vi "Read.vi"(8 "error in (no error)":errorcluster, 11 "Keyboard in":refnum<class "Keyboard.lvclass">) -> (0 "error out":errorcluster, 1 "Velocity out":dbl, 2 "Direction out":cluster{dbl, dbl}, 4 "Stop?":bool, 5 "Boost?":bool)   [LabVIEW 2024, in "Keyboard.lvclass"]
doc: "MIT Licence\nCopyright (c) 2024 David Grollier"
uses:
  Keyboard.lvclass
  Input Device.lvclass/Input Device.ctl
  Keyboard.lvclass/Keyboard.ctl
  <vilib>/Utility/error.llb/Error Cluster From Error Code.vi
  <vilib>/ErrorRing/Error Ring.xnode
  Input Device.lvclass
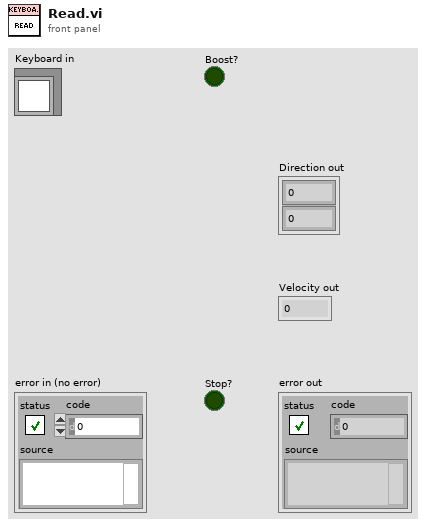
[diagram p1: front panel]
types:
  T1 = cluster{"Keyboard Registration Refnum":refnum<event-registration>, "Stop Event Registration Refnum out":refnum<event-registration>}
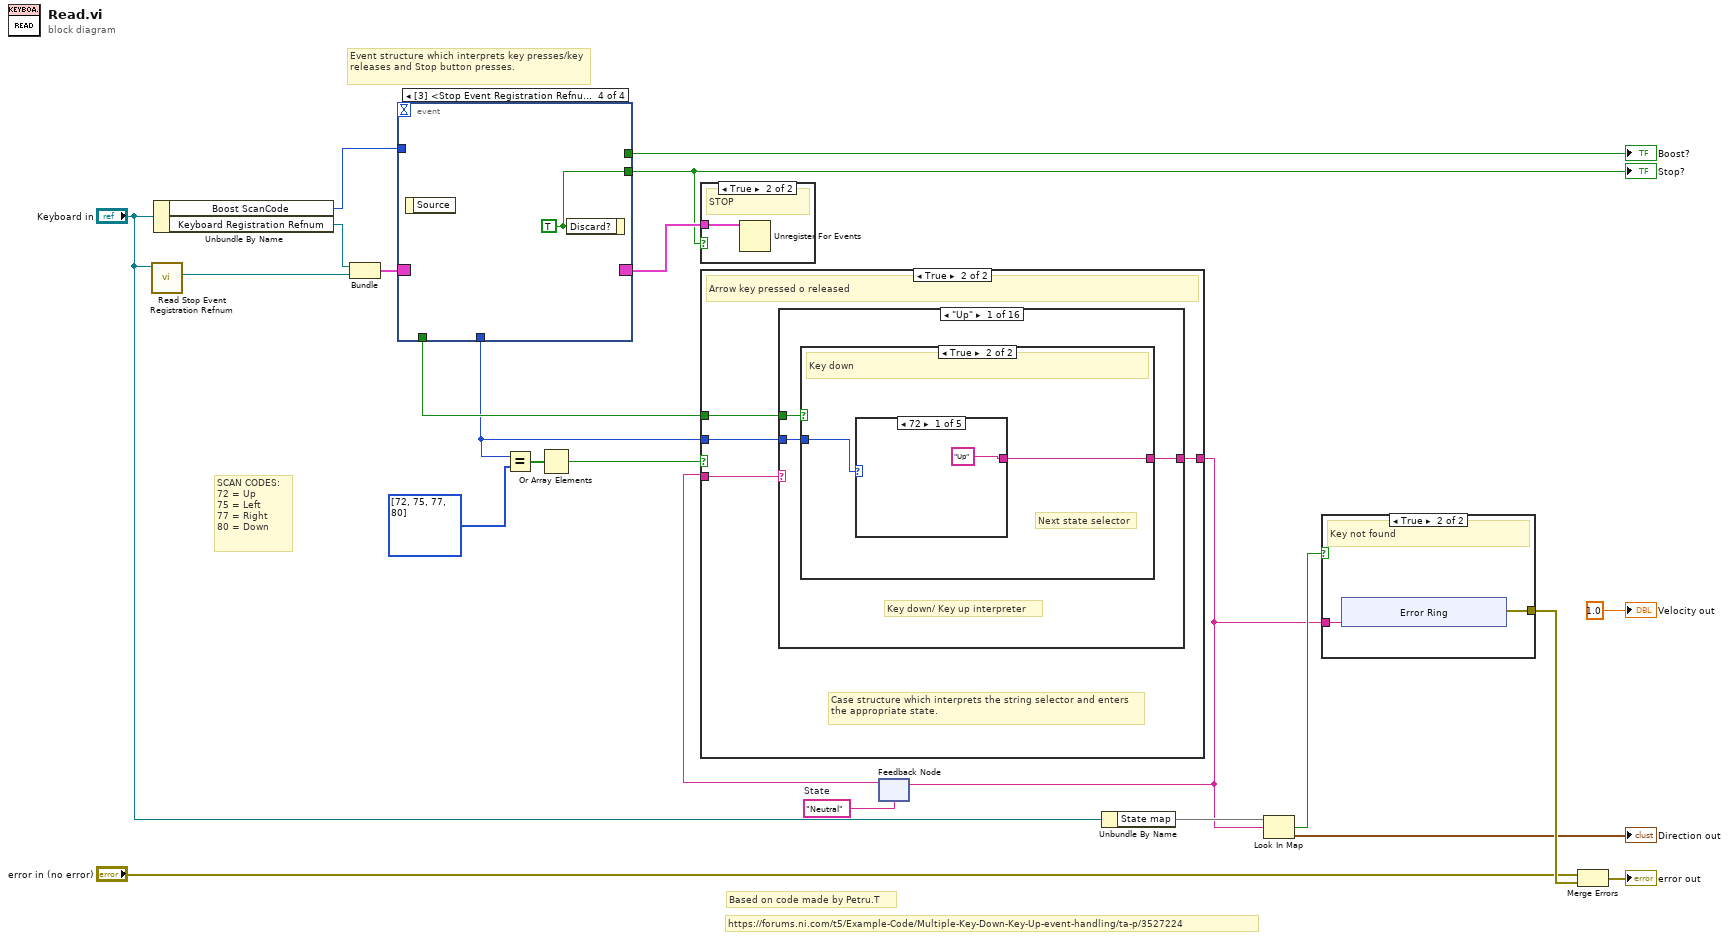
[diagram p0: block diagram]
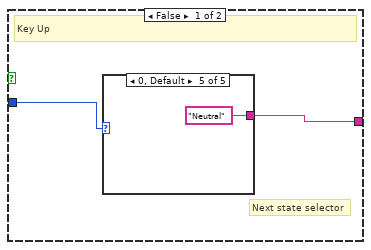
[diagram p5: hidden frame]
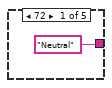
[diagram p6: hidden frame]
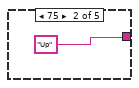
[diagram p7: hidden frame]
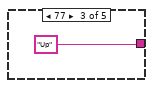
[diagram p8: hidden frame]
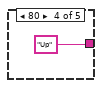
[diagram p9: hidden frame]
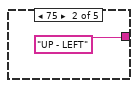
[diagram p10: hidden frame]
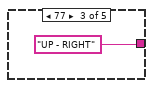
[diagram p11: hidden frame]
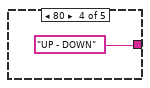
[diagram p12: hidden frame]
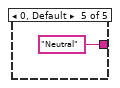
[diagram p13: hidden frame]
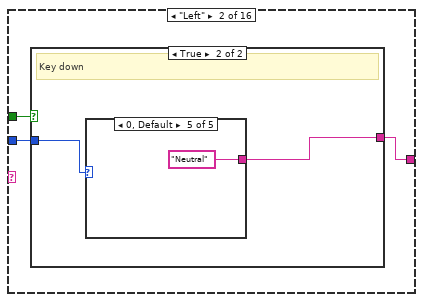
[diagram p14: hidden frame]
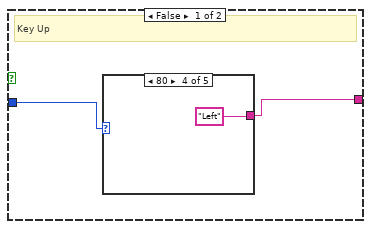
[diagram p15: hidden frame]
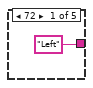
[diagram p16: hidden frame]
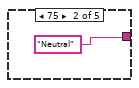
[diagram p17: hidden frame]
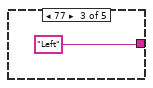
[diagram p18: hidden frame]
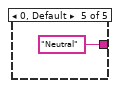
[diagram p19: hidden frame]
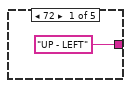
[diagram p20: hidden frame]
diagram:
  w13 = "Neutral"  # State
  # "Based on code made by Petru.T"
  # "Event structure which interprets key presses/key releases and Stop button presses."
  # "SCAN CODES:\n72 = Up\n75 = Left\n77 = Right\n80 = Down"
  # "https://forums.ni.com/t5/Example-Code/Multiple-Key-Down-Key-Up-event-handling/ta-p/3527224"
  n1 = call "Read Stop Event Registration Refnum.vi"("Input Device in"="Keyboard in") -> ("Stop Event Registration Refnum out"=w5:refnum<event-registration>)  [unwired: 10 in]
  n2 = Unbundle By Name("Keyboard in") -> ("Boost ScanCode"=w3:i16, "Keyboard Registration Refnum"=w6:refnum<event-registration>)
  n3 = Bundle("Keyboard Registration Refnum"=w6, "Stop Event Registration Refnum out"=w5) -> (w4:T1)  [unwired: 1 in]
  n4 = event shown="[3] <Stop Event Registration Refnum out.Ref FP in>: Panel Close?" {
    selector: w4 -> [_ _ _ _]
    dyn-events: [_ _ _ _] -> w14
    timeout: _ -> [_ _ _ _]
    tunnel: [_ _ TRUE w31] -> w8
    tunnel: [w24 w28 _ _] -> w10
    tunnel: [TRUE FALSE _ _] -> w23
    tunnel: w3 -> [w26 _ _ _]
    tunnel: [w25 _ _ _] -> w18
    event Key Down {
      n5 = event-data() -> ("ScanCode"=w24:i16)  [unwired: 1 in]
      n6 = Equal?(x=w26, y=w24) -> (x = y?=w25:bool)
    }
    event Key Up {
      n7 = event-data() -> ("ScanCode"=w28:i16)  [unwired: 1 in]
    }
    event User Event {
      n8 = event-data() -> ()  [unwired: 1 in, 1 out]
    }
    event Panel Close? {
      w31 = TRUE ("Discard?")
      n9 = event-data() -> ()  [unwired: 1 in, 1 out]
      n10 = event-data("Discard?"=w31) -> ()  [unwired: 1 in, 1 out]
    }
  }
  "Boost?" <- w18
  "Stop?" <- w8
  n11 = Equal?(x=w10, y=i16[] [72, 75, 77, 80]) -> (x = y?=w21:bool[])
  n12 = Or Array Elements(Boolean array=w21) -> (logical OR=w20:bool)
  n13 = case shown="True" w8 {
    tunnel: w14 -> [_ w32]
    frame False {
      # "No Stop"
    }
    frame True {
      # "STOP"
      n14 = Unregister For Events(event registration refnum=w32) -> ()  [unwired: 1 in, 1 out]
    }
  }
  n15 = feedback #1(w13) -> (w11:string)
  n16 = case shown="True" w20 {
    tunnel: w11 -> [w33 w37]
    tunnel: w23 -> [_ w36]
    tunnel: w10 -> [_ w35]
    tunnel: [w33 w34] -> w12
    frame False {
      # "Ignore any key down/key up event if it is generated by any key other than arrow keys."
      # "Key other than arrow key pressed or released"
    }
    frame True {
      # "Case structure which interprets the string selector and enters the appropriate state."
      # "Arrow key pressed o released"
      n17 = case shown="\"Up\"" w37 {
        tunnel: w36 -> [w40 w57 w74 w91 w108 w125 w142 w159 w176 w193 w210 w227 w244 w261 w278 w295]
        tunnel: w35 -> [w39 w56 w73 w90 w107 w124 w141 w158 w175 w192 w209 w226 w243 w260 w277 w294]
        tunnel: [w38 w55 w72 w89 w106 w123 w140 w157 w174 w191 w208 w225 w242 w259 w276 w293] -> w34
        frame "Up" {
          # "Key down/ Key up interpreter"
          n18 = case shown="True" w40 {
            tunnel: w39 -> [w42 w49]
            tunnel: [w41 w48] -> w38
            frame False {
              # "Next state selector"
              # "Key Up"
              n19 = case shown="0, Default" w42 {
                tunnel: ["Neutral" ("State") "Up" ("State") "Up" ("State") "Up" ("State") "Neutral" ("State")] -> w41
                frame 72 {
                }
                frame 75 {
                }
                frame 77 {
                }
                frame 80 {
                }
                frame 0, Default {
                }
              }
            }
            frame True {
              # "Next state selector"
              # "Key down"
              n20 = case shown="72" w49 {
                tunnel: ["Up" ("State") "UP - LEFT" ("State") "UP - RIGHT" ("State") "UP - DOWN" ("State") "Neutral" ("State")] -> w48
                frame 72 {
                }
                frame 75 {
                }
                frame 77 {
                }
                frame 80 {
                }
                frame 0, Default {
                }
              }
            }
          }
        }
        frame "Left" {
          n21 = case shown="True" w57 {
            tunnel: w56 -> [w59 w66]
            tunnel: [w58 w65] -> w55
            frame False {
              # "Key Up"
              n22 = case shown="80" w59 {
                tunnel: ["Left" ("State") "Neutral" ("State") "Left" ("State") "Left" ("State") "Neutral" ("State")] -> w58
                frame 72 {
                }
                frame 75 {
                }
                frame 77 {
                }
                frame 80 {
                }
                frame 0, Default {
                }
              }
            }
            frame True {
              # "Key down"
              n23 = case shown="0, Default" w66 {
                tunnel: ["UP - LEFT" ("State") "Left" ("State") "LEFT - RIGHT" ("State") "LEFT - DOWN" ("State") "Neutral" ("State")] -> w65
                frame 72 {
                }
                frame 75 {
                }
                frame 77 {
                }
                frame 80 {
                }
                frame 0, Default {
                }
              }
            }
          }
        }
        frame "Right" {
          n24 = case shown="True" w74 {
            tunnel: w73 -> [w76 w83]
            tunnel: [w75 w82] -> w72
            frame False {
              # "Key Up"
              n25 = case shown="80" w76 {
                tunnel: ["Right" ("State") "Right" ("State") "Neutral" ("State") "Right" ("State") "Neutral" ("State")] -> w75
                frame 72 {
                }
                frame 75 {
                }
                frame 77 {
                }
                frame 80 {
                }
                frame 0, Default {
                }
              }
            }
            frame True {
              # "Key down"
              n26 = case shown="0, Default" w83 {
                tunnel: ["UP - RIGHT" ("State") "LEFT - RIGHT" ("State") "Right" ("State") "RIGHT - DOWN" ("State") "Neutral" ("State")] -> w82
                frame 72 {
                }
                frame 75 {
                }
                frame 77 {
                }
                frame 80 {
                }
                frame 0, Default {
                }
              }
            }
          }
        }
        frame "Down" {
          n27 = case shown="True" w91 {
            tunnel: w90 -> [w93 w100]
            tunnel: [w92 w99] -> w89
            frame False {
              # "Key Up"
              n28 = case shown="80" w93 {
                tunnel: ["Down" ("State") "Down" ("State") "Down" ("State") "Neutral" ("State") "Neutral" ("State")] -> w92
                frame 72 {
                }
                frame 75 {
                }
                frame 77 {
                }
                frame 80 {
                }
                frame 0, Default {
                }
              }
            }
            frame True {
              # "Key down"
              n29 = case shown="72" w100 {
                tunnel: ["UP - DOWN" ("State") "LEFT - DOWN" ("State") "RIGHT - DOWN" ("State") "Down" ("State") "Neutral" ("State")] -> w99
                frame 72 {
                }
                frame 75 {
                }
                frame 77 {
                }
                frame 80 {
                }
                frame 0, Default {
                }
              }
            }
          }
        }
        frame "UP - LEFT" {
          n30 = case shown="False" w108 {
            tunnel: w107 -> [w110 w117]
            tunnel: [w109 w116] -> w106
            frame False {
              # "Key Up"
              n31 = case shown="80" w110 {
                tunnel: ["Left" ("State") "Up" ("State") "UP - LEFT" ("State") "UP - LEFT" ("State") "Neutral" ("State")] -> w109
                frame 72 {
                }
                frame 75 {
                }
                frame 77 {
                }
                frame 80 {
                }
                frame 0, Default {
                }
              }
            }
            frame True {
              # "Key down"
              n32 = case shown="0, Default" w117 {
                tunnel: ["UP - LEFT" ("State") "UP - LEFT" ("State") "UP - LEFT - RIGHT" ("State") "UP - LEFT - DOWN" ("State") "Neutral" ("State")] -> w116
                frame 72 {
                }
                frame 75 {
                }
                frame 77 {
                }
                frame 80 {
                }
                frame 0, Default {
                }
              }
            }
          }
        }
        frame "UP - RIGHT" {
          n33 = case shown="True" w125 {
            tunnel: w124 -> [w127 w134]
            tunnel: [w126 w133] -> w123
            frame False {
              # "Key Up"
              n34 = case shown="0, Default" w127 {
                tunnel: ["Right" ("State") "UP - RIGHT" ("State") "Up" ("State") "UP - RIGHT" ("State") "Neutral" ("State")] -> w126
                frame 72 {
                }
                frame 75 {
                }
                frame 77 {
                }
                frame 80 {
                }
                frame 0, Default {
                }
              }
            }
            frame True {
              # "Key down"
              n35 = case shown="0, Default" w134 {
                tunnel: ["UP - RIGHT" ("State") "UP - LEFT - RIGHT" ("State") "UP - RIGHT" ("State") "UP - RIGHT - DOWN" ("State") "Neutral" ("State")] -> w133
                frame 72 {
                }
                frame 75 {
                }
                frame 77 {
                }
                frame 80 {
                }
                frame 0, Default {
                }
              }
            }
          }
        }
        frame "UP - DOWN" {
          n36 = case shown="True" w142 {
            tunnel: w141 -> [w144 w151]
            tunnel: [w143 w150] -> w140
            frame False {
              # "Key Up"
              n37 = case shown="0, Default" w144 {
                tunnel: ["Down" ("State") "UP - DOWN" ("State") "UP - DOWN" ("State") "Up" ("State") "Neutral" ("State")] -> w143
                frame 72 {
                }
                frame 75 {
                }
                frame 77 {
                }
                frame 80 {
                }
                frame 0, Default {
                }
              }
            }
            frame True {
              # "Key down"
              n38 = case shown="75" w151 {
                tunnel: ["UP - DOWN" ("State") "UP - LEFT - DOWN" ("State") "UP - RIGHT - DOWN" ("State") "UP - DOWN" ("State") "Neutral" ("State")] -> w150
                frame 72 {
                }
                frame 75 {
                }
                frame 77 {
                }
                frame 80 {
                }
                frame 0, Default {
                }
              }
            }
          }
        }
        frame "LEFT - RIGHT" {
          n39 = case shown="False" w159 {
            tunnel: w158 -> [w161 w168]
            tunnel: [w160 w167] -> w157
            frame False {
              # "Key Up"
              n40 = case shown="80" w161 {
                tunnel: ["LEFT - RIGHT" ("State") "Right" ("State") "Left" ("State") "LEFT - RIGHT" ("State") "Neutral" ("State")] -> w160
                frame 72 {
                }
                frame 75 {
                }
                frame 77 {
                }
                frame 80 {
                }
                frame 0, Default {
                }
              }
            }
            frame True {
              # "Key down"
              n41 = case shown="80" w168 {
                tunnel: ["UP - LEFT - RIGHT" ("State") "LEFT - RIGHT" ("State") "LEFT - RIGHT" ("State") "LEFT - RIGHT - DOWN" ("State") "Neutral" ("State")] -> w167
                frame 72 {
                }
                frame 75 {
                }
                frame 77 {
                }
                frame 80 {
                }
                frame 0, Default {
                }
              }
            }
          }
        }
        frame "LEFT - DOWN" {
          n42 = case shown="False" w176 {
            tunnel: w175 -> [w178 w185]
            tunnel: [w177 w184] -> w174
            frame False {
              # "Key Up"
              n43 = case shown="80" w178 {
                tunnel: ["LEFT - DOWN" ("State") "Down" ("State") "LEFT - DOWN" ("State") "Left" ("State") "Neutral" ("State")] -> w177
                frame 72 {
                }
                frame 75 {
                }
                frame 77 {
                }
                frame 80 {
                }
                frame 0, Default {
                }
              }
            }
            frame True {
              # "Key down"
              n44 = case shown="0, Default" w185 {
                tunnel: ["UP - LEFT - DOWN" ("State") "LEFT - DOWN" ("State") "LEFT - RIGHT - DOWN" ("State") "LEFT - DOWN" ("State") "Neutral" ("State")] -> w184
                frame 72 {
                }
                frame 75 {
                }
                frame 77 {
                }
                frame 80 {
                }
                frame 0, Default {
                }
              }
            }
          }
        }
        frame "RIGHT - DOWN" {
          n45 = case shown="True" w193 {
            tunnel: w192 -> [w195 w202]
            tunnel: [w194 w201] -> w191
            frame False {
              # "Key Up"
              n46 = case shown="0, Default" w195 {
                tunnel: ["RIGHT - DOWN" ("State") "RIGHT - DOWN" ("State") "Down" ("State") "Right" ("State") "Neutral" ("State")] -> w194
                frame 72 {
                }
                frame 75 {
                }
                frame 77 {
                }
                frame 80 {
                }
                frame 0, Default {
                }
              }
            }
            frame True {
              # "Key down"
              n47 = case shown="0, Default" w202 {
                tunnel: ["UP - RIGHT - DOWN" ("State") "LEFT - RIGHT - DOWN" ("State") "RIGHT - DOWN" ("State") "RIGHT - DOWN" ("State") "Neutral" ("State")] -> w201
                frame 72 {
                }
                frame 75 {
                }
                frame 77 {
                }
                frame 80 {
                }
                frame 0, Default {
                }
              }
            }
          }
        }
        frame "UP - LEFT - RIGHT" {
          n48 = case shown="True" w210 {
            tunnel: w209 -> [w212 w219]
            tunnel: [w211 w218] -> w208
            frame False {
              # "Key Up"
              n49 = case shown="0, Default" w212 {
                tunnel: ["LEFT - RIGHT" ("State") "UP - RIGHT" ("State") "UP - LEFT" ("State") "UP - LEFT - RIGHT" ("State") "Neutral" ("State")] -> w211
                frame 72 {
                }
                frame 75 {
                }
                frame 77 {
                }
                frame 80 {
                }
                frame 0, Default {
                }
              }
            }
            frame True {
              # "Key down"
              n50 = case shown="0, Default" w219 {
                tunnel: ["UP - LEFT - RIGHT" ("State") "UP - LEFT - RIGHT" ("State") "UP - LEFT - RIGHT" ("State") "UP - LEFT - RIGHT - DOWN" ("State") "Neutral" ("State")] -> w218
                frame 72 {
                }
                frame 75 {
                }
                frame 77 {
                }
                frame 80 {
                }
                frame 0, Default {
                }
              }
            }
          }
        }
        frame "UP - LEFT - DOWN" {
          n51 = case shown="True" w227 {
            tunnel: w226 -> [w229 w236]
            tunnel: [w228 w235] -> w225
            frame False {
              # "Key Up"
              n52 = case shown="80" w229 {
                tunnel: ["LEFT - DOWN" ("State") "UP - DOWN" ("State") "UP - LEFT - DOWN" ("State") "UP - LEFT" ("State") "Neutral" ("State")] -> w228
                frame 72 {
                }
                frame 75 {
                }
                frame 77 {
                }
                frame 80 {
                }
                frame 0, Default {
                }
              }
            }
            frame True {
              # "Key down"
              n53 = case shown="80" w236 {
                tunnel: ["UP - LEFT - DOWN" ("State") "UP - LEFT - DOWN" ("State") "UP - LEFT - RIGHT - DOWN" ("State") "UP - LEFT - DOWN" ("State") "Neutral" ("State")] -> w235
                frame 72 {
                }
                frame 75 {
                }
                frame 77 {
                }
                frame 80 {
                }
                frame 0, Default {
                }
              }
            }
          }
        }
        frame "UP - RIGHT - DOWN" {
          n54 = case shown="True" w244 {
            tunnel: w243 -> [w246 w253]
            tunnel: [w245 w252] -> w242
            frame False {
              # "Key Up"
              n55 = case shown="0, Default" w246 {
                tunnel: ["RIGHT - DOWN" ("State") "UP - RIGHT - DOWN" ("State") "UP - DOWN" ("State") "UP - RIGHT" ("State") "Neutral" ("State")] -> w245
                frame 72 {
                }
                frame 75 {
                }
                frame 77 {
                }
                frame 80 {
                }
                frame 0, Default {
                }
              }
            }
            frame True {
              # "Key down"
              n56 = case shown="0, Default" w253 {
                tunnel: ["UP - RIGHT - DOWN" ("State") "UP - LEFT - RIGHT - DOWN" ("State") "UP - RIGHT - DOWN" ("State") "UP - RIGHT - DOWN" ("State") "Neutral" ("State")] -> w252
                frame 72 {
                }
                frame 75 {
                }
                frame 77 {
                }
                frame 80 {
                }
                frame 0, Default {
                }
              }
            }
          }
        }
        frame "LEFT - RIGHT - DOWN" {
          n57 = case shown="False" w261 {
            tunnel: w260 -> [w263 w270]
            tunnel: [w262 w269] -> w259
            frame False {
              # "Key Up"
              n58 = case shown="80" w263 {
                tunnel: ["LEFT - RIGHT - DOWN" ("State") "RIGHT - DOWN" ("State") "LEFT - DOWN" ("State") "LEFT - RIGHT" ("State") "Neutral" ("State")] -> w262
                frame 72 {
                }
                frame 75 {
                }
                frame 77 {
                }
                frame 80 {
                }
                frame 0, Default {
                }
              }
            }
            frame True {
              # "Key down"
              n59 = case shown="80" w270 {
                tunnel: ["UP - LEFT - RIGHT - DOWN" ("State") "LEFT - RIGHT - DOWN" ("State") "LEFT - RIGHT - DOWN" ("State") "LEFT - RIGHT - DOWN" ("State") "Neutral" ("State")] -> w269
                frame 72 {
                }
                frame 75 {
                }
                frame 77 {
                }
                frame 80 {
                }
                frame 0, Default {
                }
              }
            }
          }
        }
        frame "UP - LEFT - RIGHT - DOWN" {
          n60 = case shown="False" w278 {
            tunnel: w277 -> [w280 w287]
            tunnel: [w279 w286] -> w276
            frame False {
              # "Key Up"
              n61 = case shown="80" w280 {
                tunnel: ["LEFT - RIGHT - DOWN" ("State") "UP - RIGHT - DOWN" ("State") "UP - LEFT - DOWN" ("State") "UP - LEFT - RIGHT" ("State") "Neutral" ("State")] -> w279
                frame 72 {
                }
                frame 75 {
                }
                frame 77 {
                }
                frame 80 {
                }
                frame 0, Default {
                }
              }
            }
            frame True {
              # "Key down"
              n62 = case shown="80" w287 {
                tunnel: ["UP - LEFT - RIGHT - DOWN" ("State") "UP - LEFT - RIGHT - DOWN" ("State") "UP - LEFT - RIGHT - DOWN" ("State") "UP - LEFT - RIGHT - DOWN" ("State") "Neutral" ("State")] -> w286
                frame 72 {
                }
                frame 75 {
                }
                frame 77 {
                }
                frame 80 {
                }
                frame 0, Default {
                }
              }
            }
          }
        }
        frame "Neutral", Default {
          n63 = case shown="True" w295 {
            tunnel: w294 -> [_ w298]
            tunnel: ["Neutral" ("State") w297] -> w293
            frame False {
              # "Key Up"
            }
            frame True {
              # "Next state selector"
              # "Key down"
              n64 = case shown="0, Default" w298 {
                tunnel: ["Neutral" ("State") "Up" ("State") "Left" ("State") "Right" ("State") "Down" ("State")] -> w297
                frame 0, Default {
                }
                frame 72 {
                }
                frame 75 {
                }
                frame 77 {
                }
                frame 80 {
                }
              }
            }
          }
        }
      }
    }
  }
  n65 = feedback-in #1(w12) -> ()
  n66 = Unbundle By Name("Keyboard in") -> ("State map"=w19:map{string, cluster{dbl, dbl}})
  n67 = Look In Map(map=w19, key=w12) -> (key not found?=w17:bool, value=→"Direction out":cluster{dbl, dbl})  [unwired: 1 in]
  n68 = case shown="True" w17 {
    tunnel: w12 -> [_ w305]
    tunnel: [_ w304] -> w16
    frame False {
      # "Key found"
    }
    frame True {
      # "Key not found"
      n69 = xnode "Error Ring"("parameter 0"=w305) -> ("error out"=w304:errorcluster)
    }
  }
  n70 = Merge Errors("error in (no error)", w16) -> (→"error out":errorcluster)
  "Velocity out" <- 1.0 ("Velocity out")
